vi "Find Font.vi"(8 "error in":errorcluster, 10 "Font":T1={"Bold"=enum."bold", "Italic"=enum."default", "Underline"=enum."none", "TextColor"=0, "TextSize"=-1.0, "Name"=""}, 11 "SpreadsheetDoc in":refnum<k24>) -> (0 "error out":errorcluster, 1 "FontId":i32, 2 "Font":refnum<k24>, 3 "SpreadsheetDoc out":refnum<k24>)   [LabVIEW 2021, in "Open Xml.lvlib"]
uses:
  Open Xml.lvlib
  D:/git/Open-Xml-LabVIEW/dll/DocumentFormat.OpenXml.Framework.dll
  dll/DocumentFormat.OpenXml.Framework.dll
  D:/git/Open-Xml-LabVIEW/dll/DocumentFormat.OpenXml.dll
  dll/DocumentFormat.OpenXml.dll
  Font.ctl
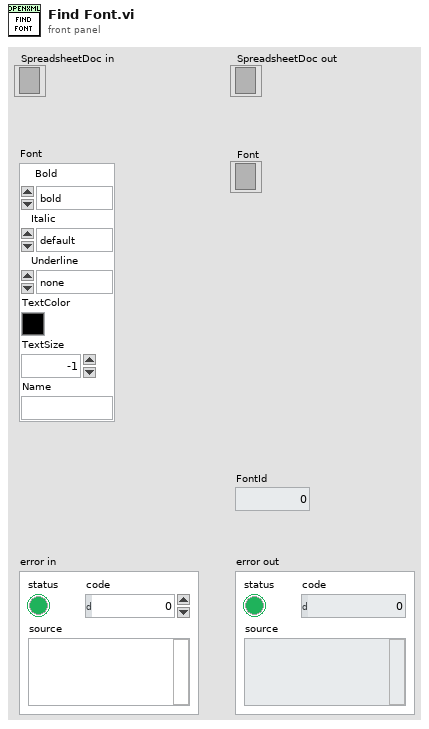
[diagram p1: front panel]
types:
  T1 = typedef "Open Xml.lvlib/Font.ctl" = cluster{"Bold":enum16{"bold", "regular", "default"}, "Italic":enum16{"italic", "regular", "default"}, "Underline":enum16{"single", "double", "singleAccounting", "doubleAccounting", "none", "default"}, "TextColor":u32, "TextSize":dbl, "Name":string}
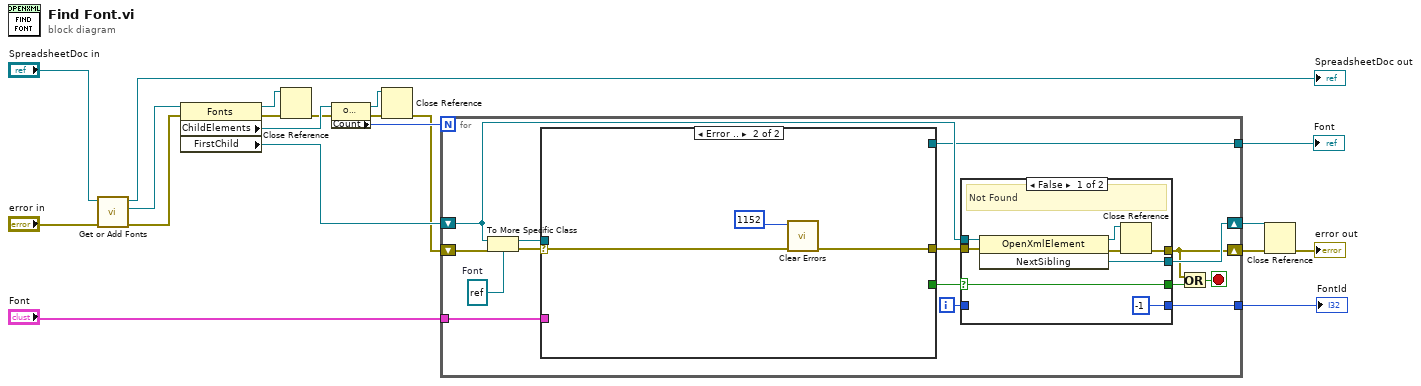
[diagram p0: block diagram]
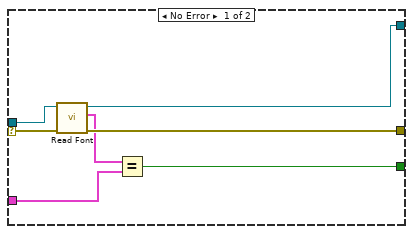
[diagram p2: hidden frame]
diagram:
  n1 = call "Get or Add Fonts.vi"("error in"="error in", "SpreadsheetDoc in"="SpreadsheetDoc in") -> ("error out"=w14:errorcluster, "Fonts"=w17:refnum<k24>, "SpreadsheetDoc out"=→"SpreadsheetDoc out":refnum<k24>)  [unwired: 7 in]
  n2 = property class="Fonts"(reference=w17, error in=w14) -> (reference out=w3:refnum<k24>, error out=w13:errorcluster, "ChildElements"=w16:refnum<k24>, "FirstChild"=w12:refnum<k24>)
  n3 = Close Reference(reference=w3, error in (no error)=w13) -> (error out=w4:errorcluster)
  n4 = property class="OpenXmlElementList"(reference=w16, error in=w4) -> (reference out=w1:refnum<k24>, error out=w11:errorcluster, "Count"=w15:i32)
  n5 = Close Reference(reference=w1, error in (no error)=w11) -> (error out=w2:errorcluster)
  n6 = for {
    N: w15 -> [_]
    shift-right: [w27] -> w7
    shift-left: w12 -> [w31]
    shift-right: [w26] -> w10
    shift-left: w2 -> [w34]
    tunnel: "Font" -> [w21]
    tunnel: [w28] -> w9
    tunnel: [w22] -> w5
    i -> [w23]
    stop <- w29 stop-if-true
    w33 = refnum<k24> refnum  # Font
    n7 = To More Specific Class(target class=w33, reference=w31, error in=w34) -> (specific class reference=w35:refnum<k24>, error out=w32:errorcluster)
    n8 = case shown="Error .." w32 {
      selector: w32 -> [w42 w45]
      tunnel: w35 -> [w41 _]
      tunnel: [w40 w44] -> w30
      tunnel: [w37 _] -> w25
      tunnel: [w36 _] -> w28
      tunnel: w21 -> [w38 _]
      frame No Error {
        n9 = call "Read Font.vi"("error in"=w42, "Font in"=w41) -> ("error out"=w40:errorcluster, "Font"=w39:T1, "Font out"=w36:refnum<k24>)  [unwired: 7 in]
        n10 = Equal?(x=w39, y=w38) -> (x = y?=w37:bool)
      }
      frame Error {
        n11 = call <vilib>:"Clear Errors.vi"("error in (no error)"=w45, "specific error code to clear (0: all)"=1152) -> ("error out"=w44:errorcluster)  [unwired: 4 in, 1 out]
      }
    }
    n12 = case shown="False" w25 {
      selector: w25 -> [w47 w55]
      tunnel: w31 -> [w53 _]
      tunnel: w30 -> [w52 w56]
      tunnel: [w51 _] -> w27
      tunnel: [w48 w56] -> w26
      tunnel: [w47 w55] -> w24
      tunnel: w23 -> [_ w54]
      tunnel: [-1 w54] -> w22
      frame False {
        # "Not Found"
        n13 = invoke class="OpenXmlElement" method="NextSibling"(reference=w53, error in=w52) -> (reference out=w50:refnum<k24>, error out=w49:errorcluster, "NextSibling"=w51:refnum<k24>)  [unwired: 1 in]
        n14 = Close Reference(reference=w50, error in (no error)=w49) -> (error out=w48:errorcluster)
      }
      frame True {
        # "Found"
      }
    }
    n15 = Or(x=w26, y=w24) -> (x .or. y?=w29:bool)
  }
  "Font" <- w9
  "FontId" <- w5
  n16 = Close Reference(reference=w7, error in (no error)=w10) -> (error out=→"error out":errorcluster)
